vi "host.sandbox.vi"() -> ()   [LabVIEW 2022 SP3]
panel:
  out "My Cluster Out":cluster{string, i32}
  in  "My Cluster":cluster{string, i32}
  out "My Array Out":i32[](array[numeric])
  in  "My Array":i32[](array[numeric])
  out "My String Out":string
  in  "My String":string
  out "error out":errorcluster
  out "tempData":variant
  in  "error in (no error)":errorcluster
  out "SampleInterval":dbl
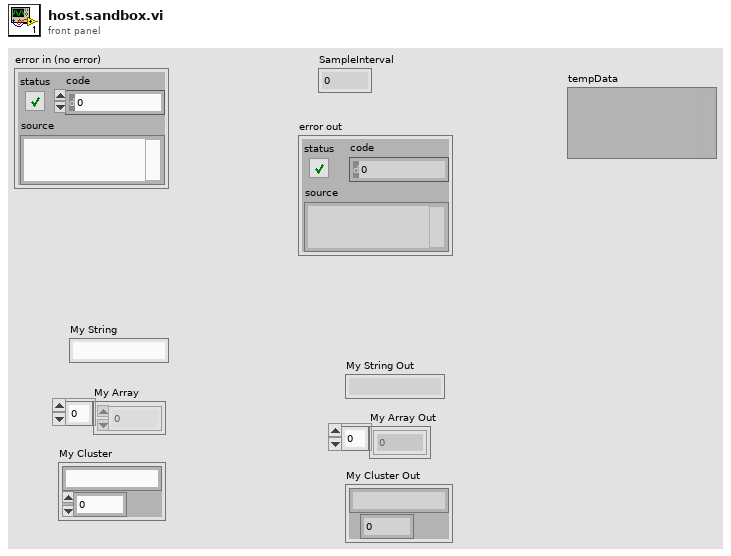
[diagram p1: front panel]
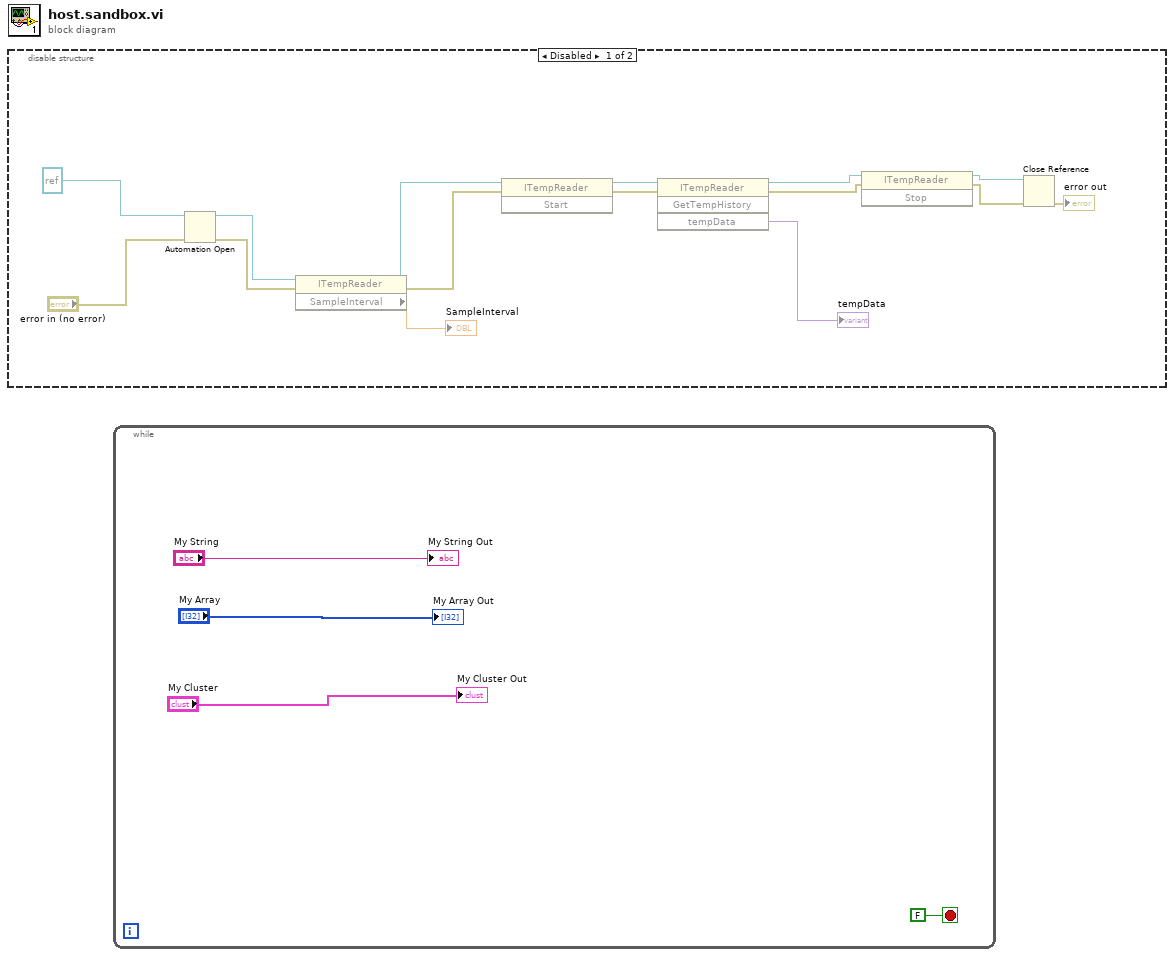
[diagram p0: block diagram]
diagram:
  n1 = disable-structure shown="Disabled" {
    frame Disabled {
      n2 = Automation Open(error in (no error)="error in (no error)", Automation Refnum=refnum<k7> refnum ("SimpleEventsServer.ITempReader")) -> (Automation Refnum=w14:refnum<k7>, error out=w11:errorcluster)  [unwired: 2 in]
      n3 = property class="ITempReader"(reference=w14, error in=w11) -> (reference out=w9:refnum<k7>, error out=w10:errorcluster, "SampleInterval"=→"SampleInterval":dbl)
      n4 = invoke class="ITempReader" method="Start"(reference=w9, error in=w10) -> (reference out=w8:refnum<k7>, error out=w7:errorcluster)  [unwired: 1 in, 1 out]
      n5 = invoke class="ITempReader" method="GetTempHistory"(reference=w8, error in=w7) -> (reference out=w5:refnum<k7>, error out=w4:errorcluster, "tempData"=→"tempData":variant)  [unwired: 2 in, 1 out]
      n6 = invoke class="ITempReader" method="Stop"(reference=w5, error in=w4) -> (reference out=w3:refnum<k7>, error out=w2:errorcluster)  [unwired: 1 in, 1 out]
      n7 = Close Reference(reference=w3, error in (no error)=w2) -> (error out=→"error out":errorcluster)
    }
    frame Enabled {
    }
  }
  n8 = while {
    stop <- FALSE stop-if-true
    "My String Out" <- "My String"
    "My Array Out" <- "My Array"
    "My Cluster Out" <- "My Cluster"
  }
